vi "Configure Timestamp.vi"(0 "VISA resource name":refnum<visa-resource-name>, 5 "Timestamp Type (0: Relative)":u16(ring) items=["Relative", "Real Time Clock"], 9 "Reset Relative Time (False)":bool, 11 "error in (no error)":errorcluster) -> (4 "VISA resource name out":refnum<visa-resource-name>, 15 "error out":errorcluster)   [LabVIEW 2020, in "Keithley 27XX.lvlib"]
doc: "This VI configures the timestamp type. It also allows a way to reset the relative timestamp."
uses:
  Keithley 27XX.lvlib
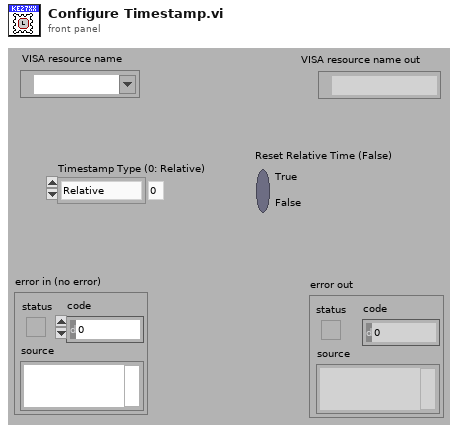
[diagram p1: front panel]
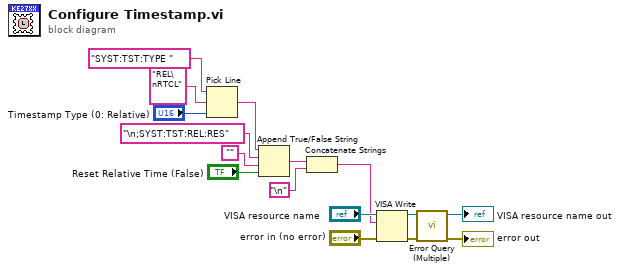
[diagram p0: block diagram]
diagram:
  n1 = Pick Line(string ("")="SYST:TST:TYPE " ("false string"), multi-line string="REL\nRTCL", line index="Timestamp Type (0: Relative)") -> (output string=w8:string)
  n2 = Append True/False String(1:"Reset Relative Time (False)", 2:"", 3:"\n;SYST:TST:REL:RES" ("false string"), 4:w8) -> (0:w3:string)
  n3 = Concatenate Strings(w3, "\n") -> (w2:string)
  n4 = VISA Write(VISA resource name="VISA resource name", write buffer=w2, error in (no error)="error in (no error)") -> (VISA resource name out=w7:refnum<visa-resource-name>, error out=w6:errorcluster)  [unwired: 1 out]
  n5 = call "Error Query (Multiple).vi"("VISA resource name"=w7, "error in (no error)"=w6) -> ("VISA resource name out"=→"VISA resource name out":refnum<visa-resource-name>, "error out"=→"error out":errorcluster)  [unwired: 10 in, 2 out]
